vi "loadChannelsInUse.vi"(6 "type":string, 8 "error in (no error)":errorcluster, 9 "device.lvclass":refnum<class "device.lvclass">, 10 "NativeXML in":refnum<class "NativeXML.lvclass">, 11 "deviceDataBase in":refnum<class "deviceDataBase.lvclass">) -> (0 "error out":errorcluster, 1 "device.lvclass out":refnum<class "device.lvclass">, 2 "NativeXML out":refnum<class "NativeXML.lvclass">, 3 "deviceDataBase out":refnum<class "deviceDataBase.lvclass">)   [LabVIEW 2009, in "Tools.lvlib" / "DatabaseHelpers.lvlib" / "deviceDataBase.lvclass"]
uses:
  deviceDataBase.lvclass
  NativeXML/NativeXML.lvclass
  Database Objects/device/device.lvclass
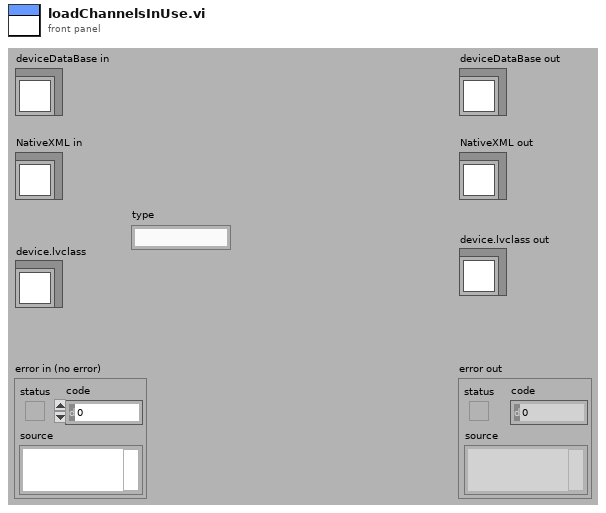
[diagram p1: front panel]
types:
  T1 = cluster{i32, "Value":string, "result string":string}
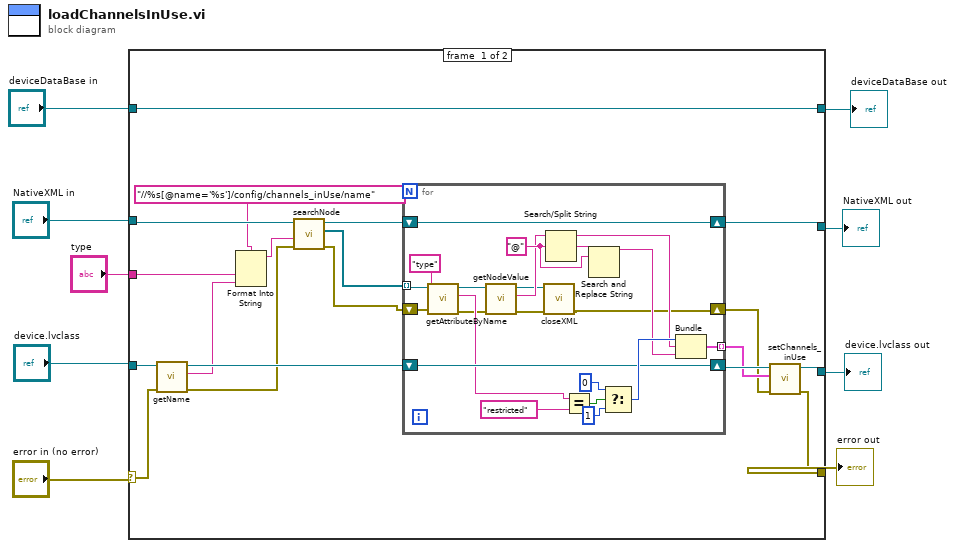
[diagram p0: block diagram]
diagram:
  n1 = case shown="No Error" "error in (no error)" {
    selector: "error in (no error)" -> [w16 w52]
    tunnel: [w24 w52] -> w8
    tunnel: [w28 w51] -> w6
    tunnel: "deviceDataBase in" -> [w28 w51]
    tunnel: "NativeXML in" -> [w20 _]
    tunnel: "device.lvclass" -> [w18 _]
    tunnel: [w23 _] -> w4
    tunnel: [w22 _] -> w3
    tunnel: "type" -> [w12 _]
    frame #0 {
      n2 = call "getName.vi"("error in (no error)"=w16, "device.lvclass in"=w18) -> ("error out"=w15:errorcluster, "name"=w13:string, "device.lvclass out"=w17:refnum<class "device.lvclass">)  [unwired: 7 in]
      n3 = Format Into String(format string="//%s[@name='%s']/config/channels_inUse/name", w12, w13) -> (resulting string=w10:string)  [unwired: 2 in, 1 out]
      n4 = call "searchNode.vi"("error in (no error)"=w15, "searchXPath"=w10, "NativeXML in"=w20) -> ("error out"=w19:errorcluster, "nodeArray"=w11:refnum<class "NativeXML.lvclass">[], "NativeXML out"=w21:refnum<class "NativeXML.lvclass">)  [unwired: 6 in]
      n5 = for {
        tunnel: w11 -> [w37] mode=indexing
        shift-right: [w29] -> w25
        shift-left: w19 -> [w38]
        shift-right: [w41] -> w27
        shift-left: w17 -> [w41]
        tunnel: [w40] -> w26 mode=indexing
        shift-right: [w39] -> w23
        shift-left: w21 -> [w39]
        w44 = "@"
        n6 = call "getAttributeByName.vi"("error in (no error)"=w38, "name"="type", "NativeXML in"=w37) -> ("error out"=w33:errorcluster, "Attribute String"=w35:string, "NativeXML out"=w34:refnum<class "NativeXML.lvclass">)  [unwired: 6 in]
        n7 = call "getNodeValue.vi"("error in (no error)"=w33, "NativeXML in"=w34) -> ("error out"=w31:errorcluster, "Value"=w32:string, "NativeXML out"=w30:refnum<class "NativeXML.lvclass">)  [unwired: 7 in]
        n8 = call "closeXML.vi"("error in (no error)"=w31, "NativeXML in"=w30) -> ("error out"=w29:errorcluster)  [unwired: 9 in]
        n9 = Search/Split String(string=w32, search string/char (-)=w44) -> (substring before match=w43:string, match + rest of string=w45:string)  [unwired: 1 in, 1 out]
        n10 = Equal?(x=w35, y="restricted") -> (x = y?=w50:bool)
        n11 = Search and Replace String(input string=w45, search string=w44) -> (result string=w42:string)  [unwired: 6 in, 3 out]
        n12 = Select(t=0, s=w50, f=1) -> (s? t:f=w46:i32)
        n13 = Bundle(w46, "Value"=w43, "result string"=w42) -> (w40:T1)  [unwired: 1 in]
      }
      n14 = call "setChannels_inUse.vi"("error in (no error)"=w25, "channels_inUse"=w26, "device.lvclass in"=w27) -> ("error out"=w24:errorcluster, "device.lvclass out"=w22:refnum<class "device.lvclass">)  [unwired: 7 in]
    }
    frame #1 {
    }
  }
  "error out" <- w8
  "deviceDataBase out" <- w6
  "NativeXML out" <- w4
  "device.lvclass out" <- w3
